vi "数组排序.vi"(10 "需要排列数据":string[][](array[string]), 11 "总数据":string[][](array[string])) -> (3 "完成后数据":string[][](array[string]))   [LabVIEW 2013]
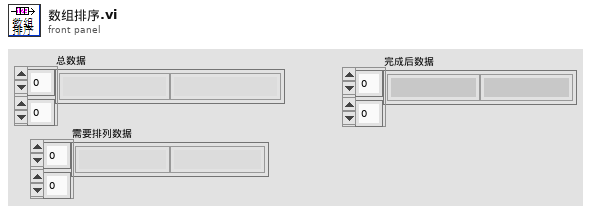
[diagram p1: front panel]
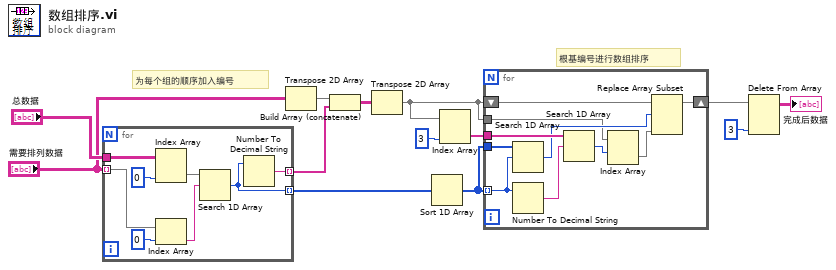
[diagram p0: block diagram]
diagram:
  # "根基编号进行数组排序"
  # "为每个组的顺序加入编号"
  n1 = for {
    tunnel: "需要排列数据" -> [w21] mode=indexing
    tunnel: "总数据" -> [w19]
    tunnel: [w15] -> w12 mode=indexing
    tunnel: [w14] -> w9 mode=indexing
    n2 = Index Array(array=w19, index (col)=0 ("禁用的索引 (列)")) -> (element=w17:string[])  [unwired: 1 in]
    n3 = Index Array(array=w21, index=0 ("索引")) -> (element=w16:string)
    n4 = Search 1D Array(1D array=w17, element=w16) -> (index of element=w14:i32)  [unwired: 1 in]
    n5 = Number To Decimal String(number=w14) -> (decimal integer string=w15:string)  [unwired: 1 in]
  }
  n6 = Transpose 2D Array(2D array="需要排列数据") -> (transposed array=w10:string[][])
  n7 = Build Array (concatenate)(w10, w12) -> (w8:string[][])
  n8 = Transpose 2D Array(2D array=w8) -> (transposed array=w5:string[][])
  n9 = Sort 1D Array(array=w9) -> (sorted array=w4:i32[])
  n10 = Index Array(array=w5, index (col)=3 ("禁用的索引 (列)")) -> (element=w6:string[])  [unwired: 1 in]
  n11 = for {
    tunnel: w4 -> [w29] mode=indexing
    tunnel: w4 -> [w31]
    tunnel: w6 -> [w30]
    shift-right: [w24] -> w3
    shift-left: w5 -> [w22]
    tunnel: w5 -> [w23]
    n12 = Search 1D Array(1D array=w31, element=w29) -> (index of element=w27:i32)  [unwired: 1 in]
    n13 = Number To Decimal String(number=w29) -> (decimal integer string=w28:string)  [unwired: 1 in]
    n14 = Search 1D Array(1D array=w30, element=w28) -> (index of element=w26:i32)  [unwired: 1 in]
    n15 = Index Array(array=w23, index (row)=w26) -> (element=w25:string[])  [unwired: 1 in]
    n16 = Replace Array Subset(array=w22, new element=w25, index (row)=w27) -> (w24:string[][])  [unwired: 1 in]
  }
  n17 = Delete From Array(array=w3, index (col)=3 ("禁用的索引 (列)")) -> (array with subset deleted=→"完成后数据":string[][])  [unwired: 2 in, 1 out]
